vi "fpga_init.vi"(11 "FPGA name":T1 caption="RIO Device") -> (0 "error out":errorcluster, 3 "FPGA VI Reference Out":refnum<k20>)   [LabVIEW 2014]
doc: "Init FPGA and Adapter Module. Run checks on Adapter module and setup DMA, used to transfer data from FPGA to Host PC."
uses:
  <vilib>/userdefined/High Color/nirio_resource_hc.ctl
  Controls/foga_init_state.ctl
  <vilib>/FPGAPlugInAG/PXIe-7962R/niLvFpga_Open_PXIe-7962R.vi
  <vilib>/rvi/interface/common/dynamic/niFpgaDynamicAddResources.vi
  <vilib>/LabVIEW Targets/FPGA/FlexRIO/CustomFPGAMethods/79XXR_Method_IOModuleStatusImpl.vi
  <vilib>/Utility/error.llb/Error Cluster From Error Code.vi
  <vilib>/rvi/errors/niLvFpgaAdjustHostInterfaceError.vi
  <vilib>/rvi/interface/common/niFpgaWaitOnOcc.vi
  <vilib>/rvi/interface/nirviOpenFPGA/nirviOpenFPGA.xnode
  FPGA Bitfiles/MochiFPGAControl_FPGATarget_pxie7962fpga_vH47uBXjtQs.lvbitx
  <vilib>/rvi/interface/nirviMethod/nirviMethod.xnode
  <vilib>/rvi/interface/nirviReadWriteControl/nirviReadWriteControl.xnode
  <vilib>/rvi/errors/niLvFpgaMergeErrorWithErrorCode.vi
  NiFpgaLv.dll
  <vilib>/rvi/interface/Simulation/niFpgaSimulationCallBeginRW.vi
  <vilib>/FPGAPlugInAG/Dynamic/niLvFpga_ConfigureFifo_Dynamic.vi
  <vilib>/FPGAPlugInAG/Dynamic/niLvFpga_StartFifo_Dynamic.vi
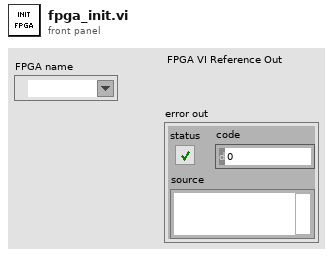
[diagram p1: front panel]
types:
  T1 = typedef "nirio_resource_hc.ctl" = tag
  T2 = typedef "foga_init_state.ctl" = enum16{"check IO module", "init IO module", "configure & start DMA"}
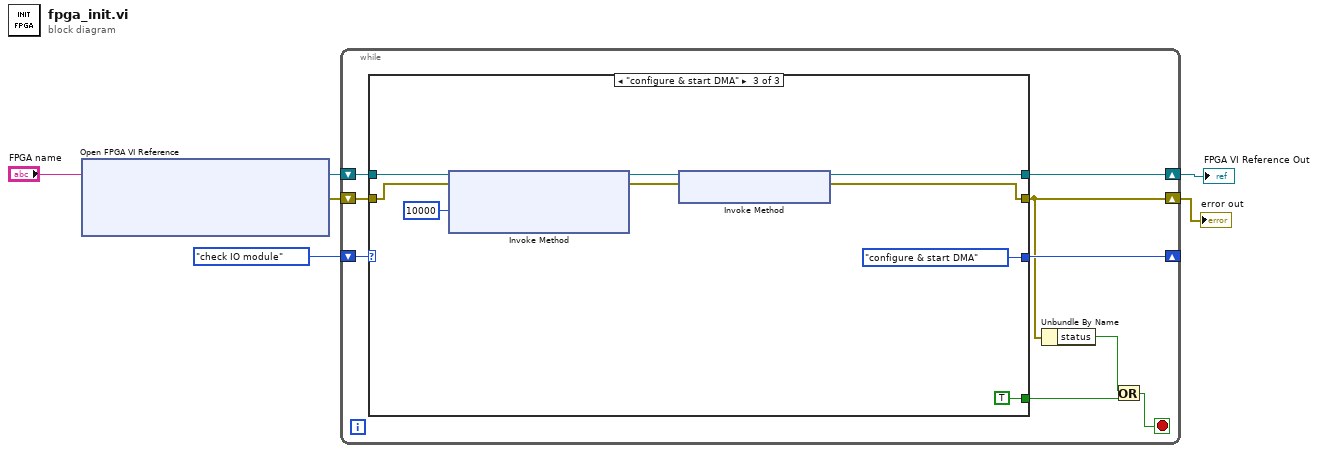
[diagram p0: block diagram]
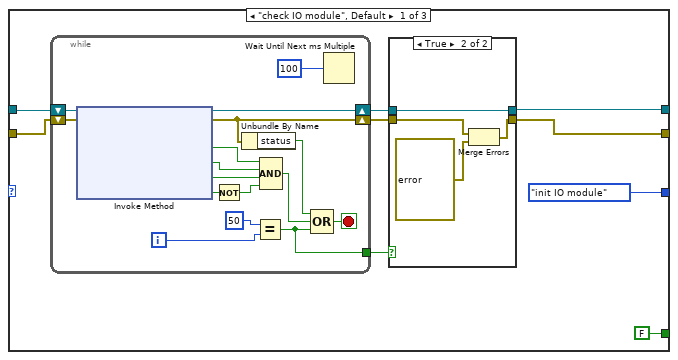
[diagram p2: hidden frame]
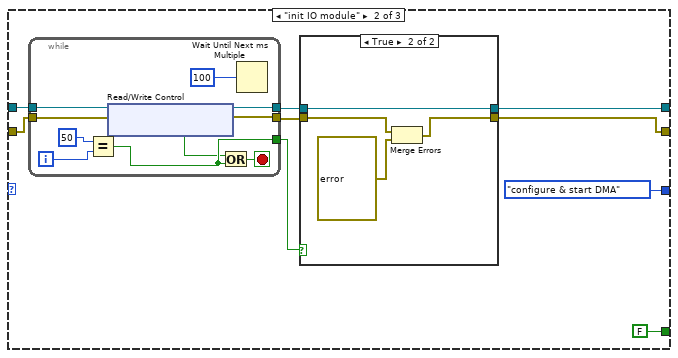
[diagram p4: hidden frame]
diagram:
  n1 = xnode "Open FPGA VI Reference"("resource name"="FPGA name") -> ("FPGA VI Reference Out"=w5:refnum<k20>, "error out"=w4:errorcluster)  [unwired: 1 in]
  n2 = while {
    shift-right: [w11] -> w1
    shift-left: w5 -> [w15]
    shift-right: [w10] -> w2
    shift-left: w4 -> [w13]
    shift-right: [w12] -> _
    shift-left: foga_init_state."check IO module" ("FPGA init state") -> [w14]
    stop <- w7 stop-if-true
    n3 = case shown="\"configure & start DMA\"" w14 {
      tunnel: w15 -> [w18 w52 w77]
      tunnel: w13 -> [w17 w51 w76]
      tunnel: [foga_init_state."init IO module" ("FPGA init state") foga_init_state."configure & start DMA" ("FPGA init state") foga_init_state."configure & start DMA" ("FPGA init state")] -> w12
      tunnel: [w20 w50 w75] -> w11
      tunnel: [w19 w49 w74] -> w10
      tunnel: [FALSE FALSE TRUE] -> w8
      frame "check IO module", Default {
        n4 = while {
          shift-right: [w37] -> w24
          shift-left: w17 -> [w45]
          shift-right: [w44] -> w22
          shift-left: w18 -> [w46]
          tunnel: [w33] -> w23
          i -> [w39]
          stop <- w34 stop-if-true
          n5 = xnode "Invoke Method"("FPGA VI Reference In"=w46, "error in"=w45) -> ("FPGA VI Reference Out"=w44:refnum<k20>, "error out"=w37:errorcluster, "IO Module Present?"=w43:bool, "Power Enabled?"=w42:bool, "IO Enabled?"=w41:bool, "IO Module Mismatch?"=w32:bool)
          n6 = Not(x=w32) -> (.not. x?=w31:bool)
          n7 = Unbundle By Name(w37) -> ("status"=w36:bool)
          n8 = Equal?(x=50, y=w39) -> (x = y?=w33:bool)
          n9 = Compound Arithmetic op=AND(w43, w42, w41, w31) -> (w35:bool)
          n10 = Compound Arithmetic op=OR(w36, w35, w33) -> (w34:bool)
          n11 = Wait Until Next ms Multiple(millisecond multiple=u32 100) -> ()  [unwired: 1 out]
        }
        n12 = case shown="True" w23 {
          tunnel: w24 -> [w25 w29]
          tunnel: [w25 w28] -> w19
          tunnel: w22 -> [w26 w27]
          tunnel: [w26 w27] -> w20
          frame False {
          }
          frame True {
            n13 = Merge Errors(w29, errorcluster {"status"=TRUE, "code"=-1, "source"="The IO Module was not present, powered, or the IO were not enabled.  Verify the NI 5752 is securly connected and try again."} ("error in")) -> (w28:errorcluster)
          }
        }
      }
      frame "init IO module" {
        n14 = while {
          tunnel: w52 -> [w66]
          tunnel: [w63] -> w54
          tunnel: [w64] -> w53
          tunnel: [w67] -> w55
          tunnel: w51 -> [w65]
          i -> [w70]
          stop <- w68 stop-if-true
          n15 = Equal?(x=50, y=w70) -> (x = y?=w67:bool)
          n16 = xnode "Read/Write Control"("FPGA VI Reference In"=w66, "error in"=w65) -> ("FPGA VI Reference Out"=w63:refnum<k20>, "error out"=w64:errorcluster, "IO Module Init Done"=w62:bool)
          n17 = Or(x=w62, y=w67) -> (x .or. y?=w68:bool)
          n18 = Wait Until Next ms Multiple(millisecond multiple=u32 100) -> ()  [unwired: 1 out]
        }
        n19 = case shown="True" w55 {
          tunnel: w53 -> [w56 w60]
          tunnel: [w56 w59] -> w49
          tunnel: w54 -> [w57 w58]
          tunnel: [w57 w58] -> w50
          frame False {
          }
          frame True {
            n20 = Merge Errors(w60, errorcluster {"status"=TRUE, "code"=-1, "source"="The IO Module CLIP was not ready. If you are using any external clocks, make sure they are connected and within the supported specifications."} ("error in")) -> (w59:errorcluster)
          }
        }
      }
      frame "configure & start DMA" {
        n21 = xnode "Invoke Method"("FPGA VI Reference In"=w77, "error in"=w76, "Requested Depth"=u32 10000) -> ("FPGA VI Reference Out"=w79:refnum<k20>, "error out"=w78:errorcluster)  [unwired: 1 out]
        n22 = xnode "Invoke Method"("FPGA VI Reference In"=w79, "error in"=w78) -> ("FPGA VI Reference Out"=w75:refnum<k20>, "error out"=w74:errorcluster)
      }
    }
    n23 = Unbundle By Name(w10) -> ("status"=w9:bool)
    n24 = Or(x=w9, y=w8) -> (x .or. y?=w7:bool)
  }
  "error out" <- w2
  "FPGA VI Reference Out" <- w1
